vi "公式节点.vi"() -> ()   [LabVIEW 2017]
panel:
  out "XY Graph":cluster{"Y":dbl[], "Y":dbl[]}[](graph)
  in  "d":dbl
  in  "R":dbl
  in  "r":dbl
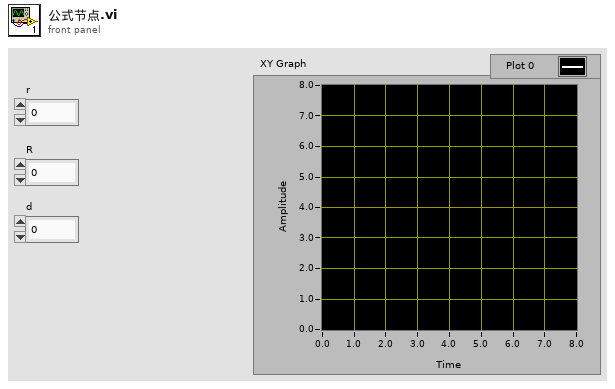
[diagram p1: front panel]
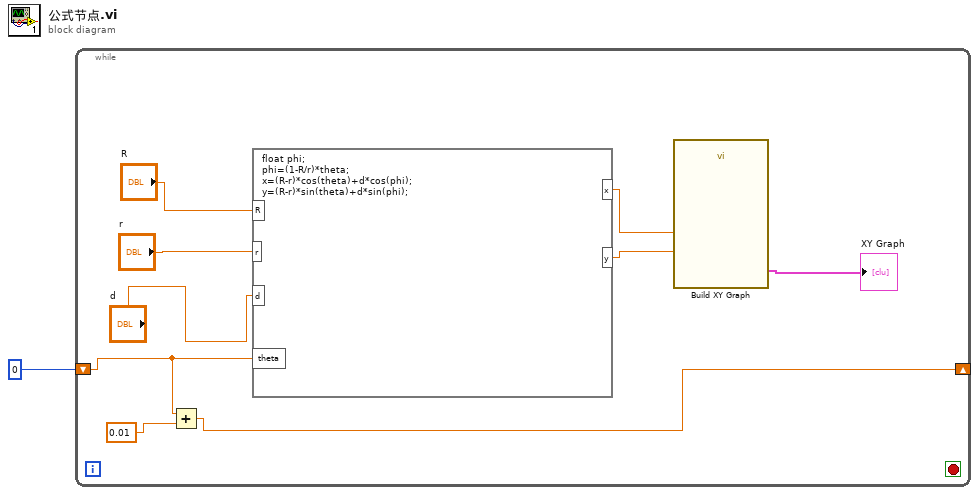
[diagram p0: block diagram]
diagram:
  n1 = while {
    shift-right: [w5] -> _
    shift-left: 0 -> [w6]
    stop <- _ stop-if-true
    n2 = Add(x=w6, y=0.01) -> (x+y=w5:dbl)
    n3 = formula code="float phi;\nphi=(1-R/r)*theta;\nx=(R-r)*cos(theta)+d*cos(phi);\ny=(R-r)*sin(theta)+d*sin(phi);"("R"="R", "r"="r", "d"="d", "theta"=w6) -> ("x"=w3:dbl, "y"=w2:dbl)
    n4 = call "Build XY Graph"("Y Input"=w2, "X Input"=w3) -> ("XY Graph"=→"XY Graph":cluster{"X":dbl[], "Y":dbl[]}[])  [unwired: 8 in, 1 out]
  }
